vi "Get 2-Exp Global Fit Guess Parameters v2.vi"(8 "Global Fit Parameter Info":T1, 9 "IRF":cluster{"t Array":dbl[], "Data Array":dbl[]}, 11 "Full Decays":cluster{"t Array":dbl[], "Value Array":dbl[]}[](array[cluster])) -> (2 "Initial Parameters":dbl[](array[numeric])=[-1.0, 0.0, 0.5, 0.1, 0.5, 1.0])   [LabVIEW 2021, in "Fits.lvlib"]
uses:
  Global Fit Parameters Information.ctl
  Fits.lvlib
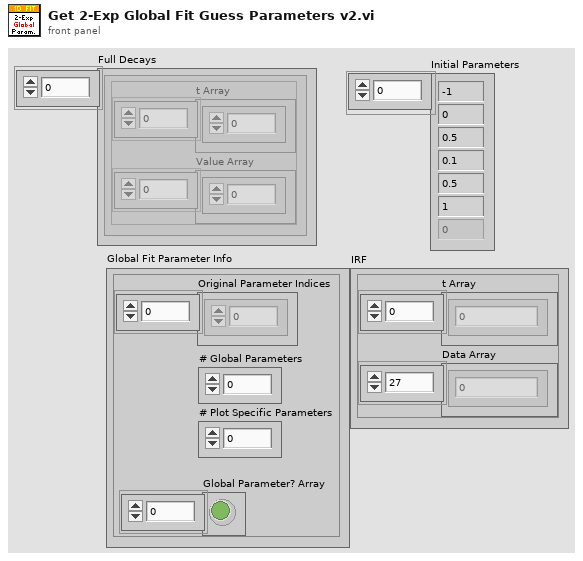
[diagram p1: front panel]
types:
  T1 = typedef "Fits.lvlib/Global Fit Parameters Information.ctl" = cluster{"Original Parameter Indices":i32[], "# Global Parameters":i32, "# Plot Specific Parameters":i32, "Global Parameter? Array":bool[]}
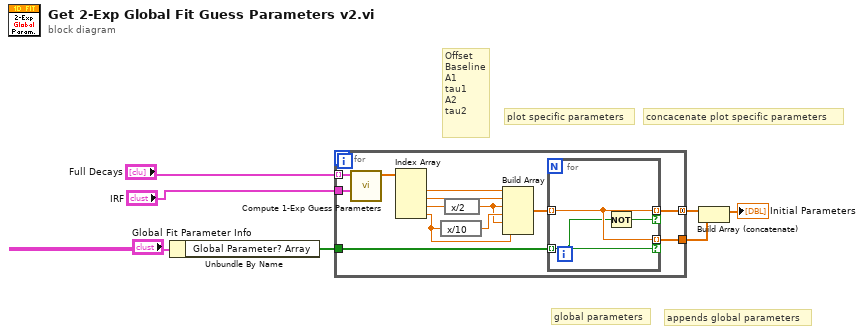
[diagram p0: block diagram]
diagram:
  # "Offset\nBaseline\nA1\ntau1\nA2\ntau2"
  # "appends global parameters"
  # "concacenate plot specific parameters"
  # "plot specific parameters"
  # "global parameters"
  n1 = Unbundle By Name("Global Fit Parameter Info") -> ("Global Parameter? Array"=w5:bool[])
  n2 = for {
    tunnel: [w19] -> w7 mode=concatenating
    tunnel: w5 -> [w20]
    tunnel: [w18] -> w3
    tunnel: "Full Decays" -> [w9] mode=indexing
    tunnel: "IRF" -> [w8]
    n3 = call "Compute 1-Exp Guess Parameters.vi"("IRF"=w8, "Decay"=w9) -> ("Guess Parameters"=w11:dbl[])  [unwired: 8 in, 1 out]
    n4 = Index Array(array=w11) -> (element #1=w17:dbl, element #2=w16:dbl, element #3=w15:dbl, element #4=w12:dbl)  [unwired: 4 in]
    n5 = expression code="x/10"(w12) -> (w14:dbl)
    n6 = expression code="x/2"(w15) -> (w13:dbl)
    n7 = Build Array(w17, w16, w13, w14, w13, w12) -> (w10:dbl[])
    n8 = for {
      tunnel: w20 -> [w22] mode=indexing
      tunnel: w10 -> [w23] mode=indexing
      tunnel: [w23] -> w18 mode=indexing if=w22
      tunnel: [w23] -> w19 mode=indexing if=w21
      n9 = Not(x=w22) -> (.not. x?=w21:bool)
    }
  }
  n10 = Build Array (concatenate)(w7, w3) -> (→"Initial Parameters":dbl[])
